vi "Get Experiments.vi"(7 "search string":string, 8 "error in (no error)":errorcluster, 9 "offset (0)":u32, 10 "limit (15)":u32=15, 11 "eLab in":refnum<class "PL eLabFTW Client.lvclass">) -> (0 "error out":errorcluster, 2 "experiments":T1(array[cluster]) {"last comment"."datetime" format="%<%X\n%x>T"; "last change"."datetime" format="%<%X\n%x>T"; "start datetime" format="%<%X\n%x>T"}, 3 "eLab out":refnum<class "PL eLabFTW Client.lvclass">)   [LabVIEW 2015, in "PL eLabFTW Client.lvclass"]
doc: "Gets experiments. Limit, offset and search string can be used to narrow down the output."
uses:
  PL eLabFTW Client.lvclass
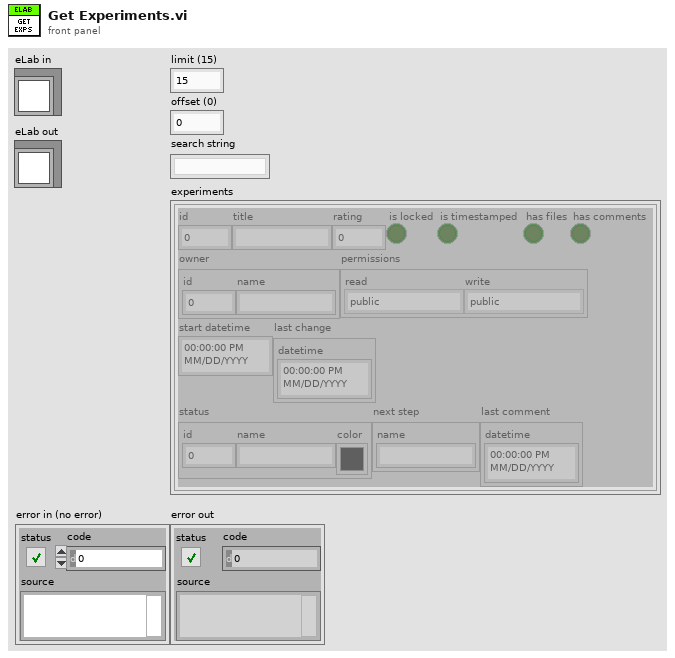
[diagram p1: front panel]
types:
  T1 = cluster{"id":u32, "title":string, "rating":u32, "is locked":bool, "is timestamped":bool, "has files":bool, "has comments":bool, "owner":cluster{"id":u32, "name":string}, "permissions":cluster{"read":enum16{"public", "organization", "team", "owner and admins", "owner"}, "write":enum16{"public", "organization", "team", "owner and admins", "owner"}}, "start datetime":timestamp, "last change":cluster{"datetime":timestamp}, "status":cluster{"id":u32, "name":string, "color":u32}, "next step":cluster{"name":string}, "last comment":cluster{"datetime":timestamp}}[]
  T2 = cluster{"id":string, "title":string, "date":string, "category":string, "rating":string, "userid":string, "locked":string, "canread":string, "canwrite":string, "lastchange":string, "up_item_id":string, "has_attachment":string, "next_step":string, "category_id":string, "color":string, "fullname":string, "recent_comment":string, "has_comment":string, "timestamped":string}[]
  T3 = cluster{"id":u32, "title":string, "rating":u32, "is locked":bool, "is timestamped":bool, "has files":bool, "has comments":bool, "owner":cluster{"id":u32, "name":string}, "permissions":cluster{"read":enum16{"public", "organization", "team", "owner and admins", "owner"}, "write":enum16{"public", "organization", "team", "owner and admins", "owner"}}, "start datetime":timestamp, "last change":cluster{"datetime":timestamp}, "status":cluster{"id":u32, "name":string, "color":u32}, "next step":cluster{"name":string}, "last comment":cluster{"datetime":timestamp}}
  T4 = enum16{"public", "organization", "team", "owner and admins", "owner"}
  T5 = cluster{"id":i32, "title":i32, "date":i32, "category":i32, "rating":i32, "userid":i32, "locked":i32, "canread":i32, "canwrite":i32, "lastchange":i32, "up_item_id":i32, "has_attachment":i32, "next_step":i32, "category_id":i32, "color":i32, "fullname":i32, "recent_comment":i32, "has_comment":i32, "timestamped":i32}
  T6 = cluster{"id":bool, "title":bool, "date":bool, "category":bool, "rating":bool, "userid":bool, "locked":bool, "canread":bool, "canwrite":bool, "lastchange":bool, "up_item_id":bool, "has_attachment":bool, "next_step":bool, "category_id":bool, "color":bool, "fullname":bool, "recent_comment":bool, "has_comment":bool, "timestamped":bool}
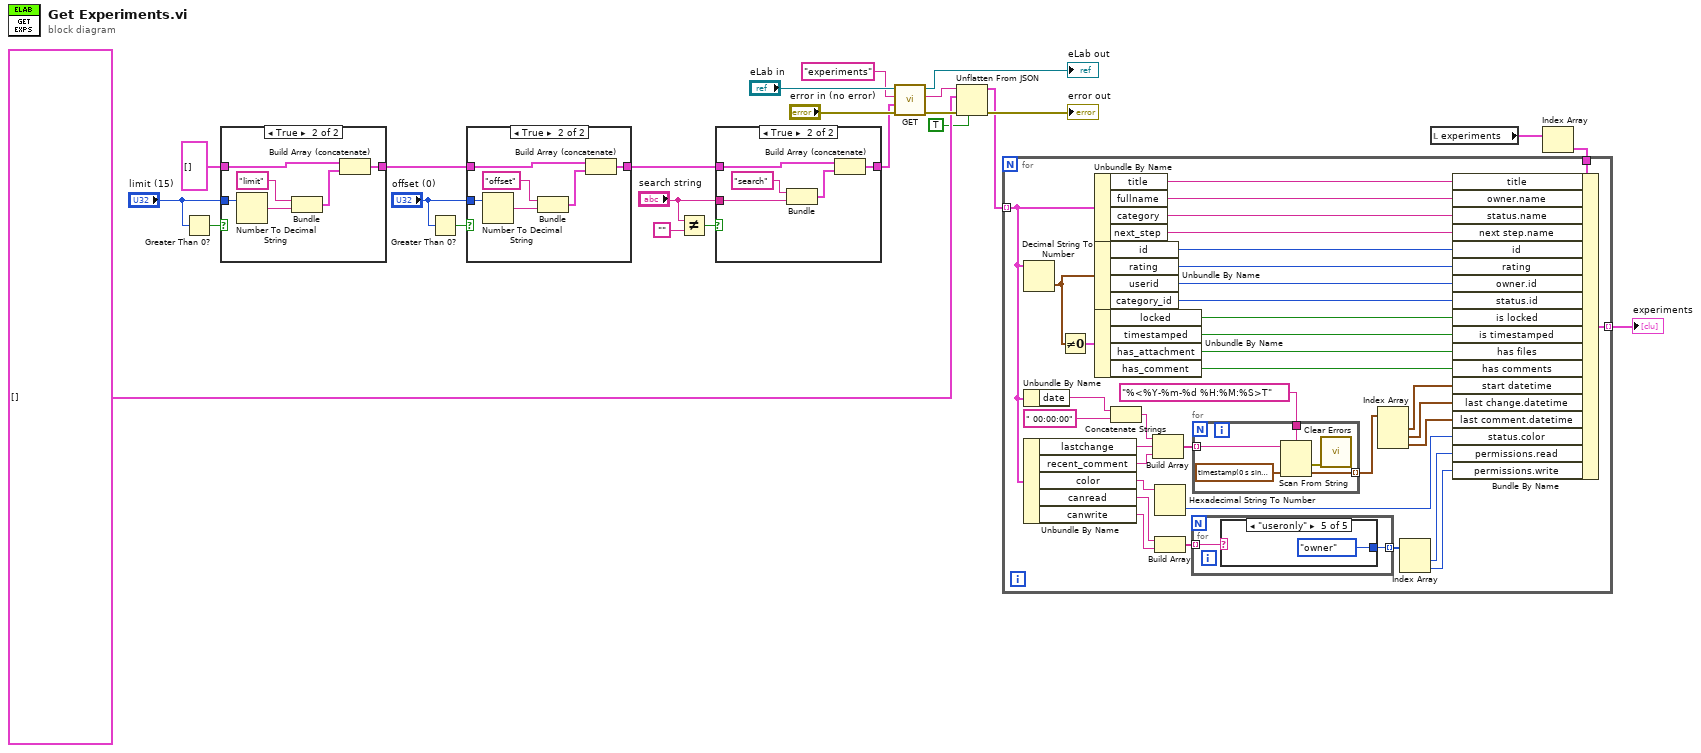
[diagram p0: block diagram]
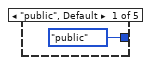
[diagram p2: hidden frame]
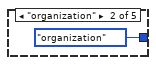
[diagram p3: hidden frame]
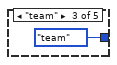
[diagram p4: hidden frame]
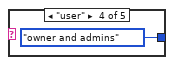
[diagram p5: hidden frame]
diagram:
  n1 = Greater Than 0?(x="limit (15)") -> (x > 0?=w17:bool)
  n2 = case shown="True" w17 {
    tunnel: "limit (15)" -> [_ w31]
    tunnel: [w25 w27] -> w12
    tunnel: cluster{string, string}[] [] -> [w25 w26]
    frame False {
    }
    frame True {
      n3 = Number To Decimal String(number=w31) -> (decimal integer string=w30:string)  [unwired: 1 in]
      n4 = Bundle("limit", w30) -> (w28:cluster{string, string})  [unwired: 1 in]
      n5 = Build Array (concatenate)(w26, w28) -> (w27:cluster{string, string}[])
    }
  }
  n6 = Greater Than 0?(x="offset (0)") -> (x > 0?=w14:bool)
  n7 = case shown="True" w14 {
    tunnel: "offset (0)" -> [_ w38]
    tunnel: [w32 w34] -> w10
    tunnel: w12 -> [w32 w33]
    frame False {
    }
    frame True {
      n8 = Number To Decimal String(number=w38) -> (decimal integer string=w37:string)  [unwired: 1 in]
      n9 = Bundle("offset", w37) -> (w35:cluster{string, string})  [unwired: 1 in]
      n10 = Build Array (concatenate)(w33, w35) -> (w34:cluster{string, string}[])
    }
  }
  n11 = Not Equal?(x="search string", y="") -> (x != y?=w11:bool)
  n12 = case shown="True" w11 {
    tunnel: "search string" -> [_ w40]
    tunnel: [w39 w42] -> w6
    tunnel: w10 -> [w39 w41]
    frame False {
    }
    frame True {
      n13 = Bundle("search", "search string"=w40) -> (w43:cluster{string, "search string":string})  [unwired: 1 in]
      n14 = Build Array (concatenate)(w41, w43) -> (w42:cluster{string, "search string":string}[])
    }
  }
  n15 = call "GET.vi"("error in (no error)"="error in (no error)", "parameters"=w6, "relative URL"="experiments", "eLab in"="eLab in") -> ("error out"=w20:errorcluster, "response body"=w3:string, "eLab out"=→"eLab out":refnum<class "PL eLabFTW Client.lvclass">)  [unwired: 5 in]
  n16 = Unflatten From JSON(JSON string=w3, type and defaults=T2 [], default null elements? (F)=TRUE, error in (no error)=w20) -> (value=w18:T2, error out=→"error out":errorcluster)  [unwired: 3 in]
  n17 = local read "experiments"() -> (w5:T1)
  n18 = Index Array(array=w5) -> (element=w4:T3)  [unwired: 1 in]
  n19 = for {
    tunnel: w18 -> [w50] mode=indexing
    tunnel: w4 -> [w45]
    tunnel: [w66] -> w1 mode=indexing
    n20 = Decimal String To Number(string=w50) -> (number=w72:T5)  [unwired: 2 in, 1 out]
    n21 = Unbundle By Name(w50) -> ("date"=w48:string)
    n22 = Unbundle By Name(w50) -> ("lastchange"=w64:string, "recent_comment"=w65:string, "color"=w59:string, "canread"=w57:string, "canwrite"=w56:string)
    n23 = Not Equal To 0?(x=w72) -> (x != 0?=w71:T6)
    n24 = Unbundle By Name(w50) -> ("title"=w80:string, "fullname"=w79:string, "category"=w78:string, "next_step"=w77:string)
    n25 = Unbundle By Name(w72) -> ("id"=w76:i32, "rating"=w75:i32, "userid"=w74:i32, "category_id"=w73:i32)
    n26 = Unbundle By Name(w71) -> ("locked"=w70:bool, "timestamped"=w69:bool, "has_attachment"=w68:bool, "has_comment"=w67:bool)
    n27 = Concatenate Strings(w48, " 00:00:00" ("string")) -> (w47:string)
    n28 = Build Array(w47, w64, w65) -> (w63:string[])
    n29 = Hexadecimal String To Number(string=w59) -> (number=w58:u32)  [unwired: 2 in, 1 out]
    n30 = Build Array(w57, w56) -> (w55:string[])
    n31 = for {
      tunnel: w55 -> [w82] mode=indexing
      tunnel: [w81] -> w54 mode=indexing
      n32 = case shown="\"useronly\"" w82 {
        tunnel: [T4."public" ("permissions.read") T4."organization" ("permissions.read") T4."team" ("permissions.read") T4."owner and admins" ("permissions.read") T4."owner" ("permissions.read")] -> w81
        frame "public", Default {
        }
        frame "organization" {
        }
        frame "team" {
        }
        frame "user" {
        }
        frame "useronly" {
        }
      }
    }
    n33 = for {
      tunnel: w63 -> [w90] mode=indexing
      tunnel: [w89] -> w62 mode=indexing
      tunnel: "%<%Y-%m-%d %H:%M:%S>T" ("format string") -> [w88]
      n34 = Scan From String(format string=w88, input string=w90, default 1=timestamp(0 s since 1904-01-01) ("from")) -> (error out=w92:errorcluster, output 1=w89:timestamp)  [unwired: 2 in, 2 out]
      n35 = call <vilib>:"Clear Errors.vi"("error in (no error)"=w92) -> ()  [unwired: 5 in, 2 out]
    }
    n36 = Index Array(array=w62) -> (element #1=w49:timestamp, element #2=w61:timestamp, element #3=w60:timestamp)  [unwired: 3 in]
    n37 = Index Array(array=w54) -> (element #1=w53:T4, element #2=w52:T4)  [unwired: 2 in]
    n38 = Bundle By Name(cluster=w45, "title"=w80, "owner.name"=w79, "status.name"=w78, "next step.name"=w77, "id"=w76, "rating"=w75, "owner.id"=w74, "status.id"=w73, "is locked"=w70, "is timestamped"=w69, "has files"=w68, "has comments"=w67, "start datetime"=w49, "last change.datetime"=w61, "last comment.datetime"=w60, "status.color"=w58, "permissions.read"=w53, "permissions.write"=w52) -> (w66:T3)
  }
  "experiments" <- w1
